vi "Home - Sync.vi"(6 "partialHome (F)":bool, 8 "error in (no error)":errorcluster, 11 "KST101 in":refnum<class "KST101.lvclass">) -> (0 "error out":errorcluster, 3 "KST101 out":refnum<class "KST101.lvclass">)   [LabVIEW 2016, in "Stepper Motor Controller.lvlib" / "KST101.lvclass"]
uses:
  KST101.lvclass
  KST101.lvclass/KST101.ctl
  D:/Workspace/ProCyteOne_LaserModuleAlignment/shared/Thorlabs/Kinesis/Dependencies/Thorlabs.MotionControl.KCube.StepperMotorCLI.dll
  Dependencies/Thorlabs.MotionControl.KCube.StepperMotorCLI.dll
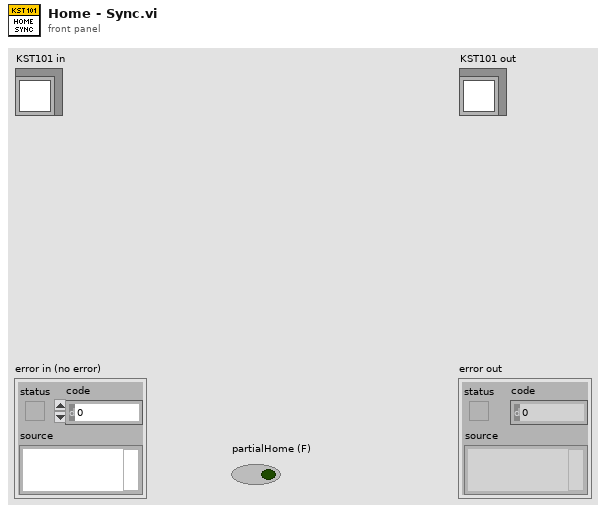
[diagram p1: front panel]
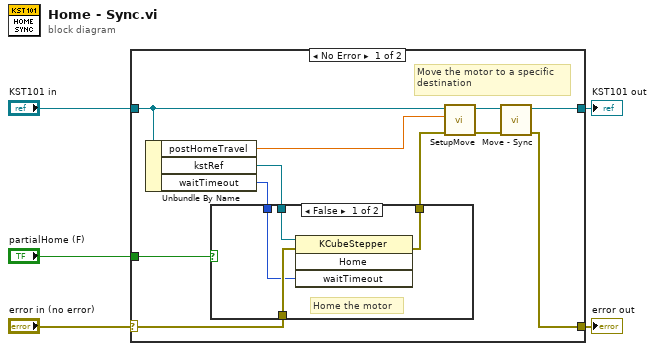
[diagram p0: block diagram]
diagram:
  n1 = case shown="No Error" "error in (no error)" {
    selector: "error in (no error)" -> [w16 w23]
    tunnel: [w10 w23] -> w4
    tunnel: [w13 w22] -> w2
    tunnel: "KST101 in" -> [w14 w22]
    tunnel: "partialHome (F)" -> [w6 _]
    frame No Error {
      # "Move the motor to a specific\ndestination"
      n2 = Unbundle By Name(w14) -> ("postHomeTravel"=w9:dbl, "kstRef"=w8:refnum<k24>, "waitTimeout"=w7:i32)
      n3 = case shown="False" w6 {
        tunnel: w16 -> [w20 w21]
        tunnel: [w19 w21] -> w11
        tunnel: w8 -> [w18 _]
        tunnel: w7 -> [w17 _]
        frame False {
          # "Home the motor"
          n4 = invoke class="KCubeStepper" method="Home"(reference=w18, error in=w20, "waitTimeout"=w17) -> (error out=w19:errorcluster)  [unwired: 1 in, 3 out]
        }
        frame True {
          # "Partial home is only moving\nto the post-home location"
        }
      }
      n5 = call-dynamic "SetupMove.vi"("error in (no error)"=w11, "moveDestination"=w9, "KST101 in"=w14) -> ("error out"=w12:errorcluster, "KST101 out"=w15:refnum<class "KST101.lvclass">)  [unwired: 7 in]
      n6 = call-dynamic "Move - Sync.vi"("error in (no error)"=w12, "KST101 in"=w15) -> ("error out"=w10:errorcluster, "KST101 out"=w13:refnum<class "KST101.lvclass">)  [unwired: 8 in]
    }
    frame Error {
    }
  }
  "error out" <- w4
  "KST101 out" <- w2
